vi "wch_labview_exp5.vi"() -> ()   [LabVIEW 2022 SP3]
uses:
  <vilib>/Analysis/NI_AALBase.lvlib
panel:
  in  "停止":bool
  in  "直流偏移 2":dbl
  in  "相位 2":dbl
  in  "幅度 2":dbl
  in  "直流偏移 1":dbl
  in  "相位 1":dbl
  in  "幅度 1":dbl
  out "相位差":dbl
  in  "采样点数":i32
  in  "采样频率":dbl
  in  "信号频率":dbl
  in  "分析方法":enum16{"过零法", "相关法", "FFT频谱分析法"}(ring)
  out "波形图":dbl[][](graph)
  # "信号 1"
  # "信号 2"
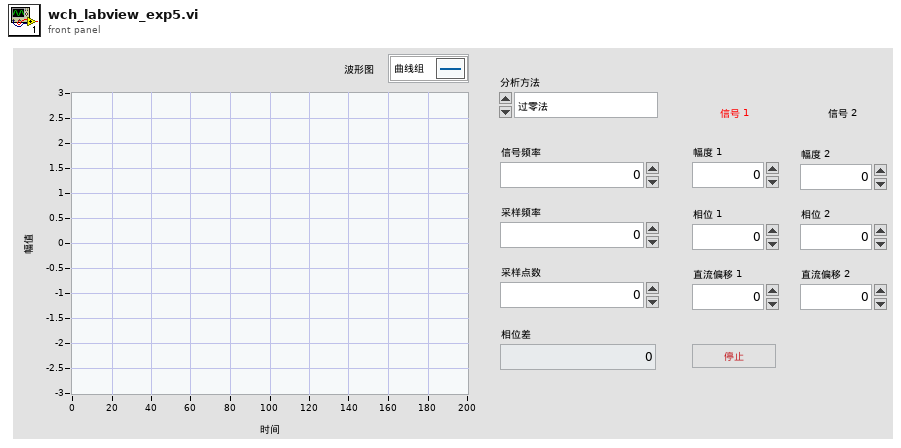
[diagram p1: front panel]
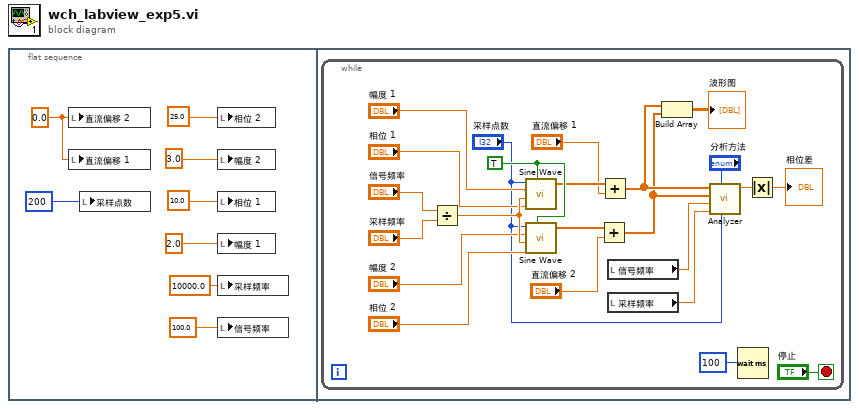
[diagram p0: block diagram]
diagram:
  n1 = flat-sequence {
    frame #0 {
      w8 = 0.0
      n2 = local write "直流偏移 2"(w8) -> ()
      n3 = local write "直流偏移 1"(w8) -> ()
      n4 = local write "采样点数"(200) -> ()
      n5 = local write "相位 2"(25.0) -> ()
      n6 = local write "幅度 2"(3.0) -> ()
      n7 = local write "相位 1"(10.0) -> ()
      n8 = local write "幅度 1"(2.0) -> ()
      n9 = local write "采样频率"(10000.0) -> ()
      n10 = local write "信号频率"(100.0) -> ()
    }
    frame #1 {
      n11 = while {
        stop <- "停止" stop-if-true
        w27 = TRUE
        n12 = Divide(x="信号频率", y="采样频率") -> (x/y=w28:dbl)
        n13 = call <vilib>:"Sine Wave.vi"("samples"="采样点数", "amplitude"="幅度 1", "frequency"=w28, "phase in"="相位 1", "reset phase"=w27) -> ("sine wave"=w21:dbl[])  [unwired: 2 out]
        n14 = call <vilib>:"Sine Wave.vi"("samples"="采样点数", "amplitude"="幅度 2", "frequency"=w28, "phase in"="相位 2", "reset phase"=w27) -> ("sine wave"=w22:dbl[])  [unwired: 2 out]
        n15 = Add(x=w22, y="直流偏移 2") -> (x+y=w16:dbl[])
        n16 = Add(x=w21, y="直流偏移 1") -> (x+y=w17:dbl[])
        n17 = local read "信号频率"() -> (w15:dbl)
        n18 = local read "采样频率"() -> (w14:dbl)
        n19 = Build Array(w17, w16) -> (→"波形图":dbl[][])
        n20 = call "Analyzer.vi"("采样点数"="采样点数", "分析方法"="分析方法", "采样频率"=w14, "信号频率"=w15, "波形 2"=w16, "波形 1"=w17) -> ("相位差"=w10:dbl)  [unwired: 5 in]
        n21 = Wait (ms)(milliseconds to wait=100) -> ()  [unwired: 1 out]
        n22 = Absolute Value(x=w10) -> (abs(x)=→"相位差":dbl)
      }
    }
  }
